vi "Parse VI Documentation String.vi"(7 "NOTE-Map":variant, 11 "Documentation":string) -> (0 "Ctrl-Doc Map":variant, 1 "Control Docs":cluster{"filtered array":string[]}[](array[cluster]), 2 "Core Doc":string, 3 "Documentation (dup)":string)   [LabVIEW 2017, in "csmdoc.lvlib"]
uses:
  csmdoc.lvlib
  Communicable State Machine.lvlib
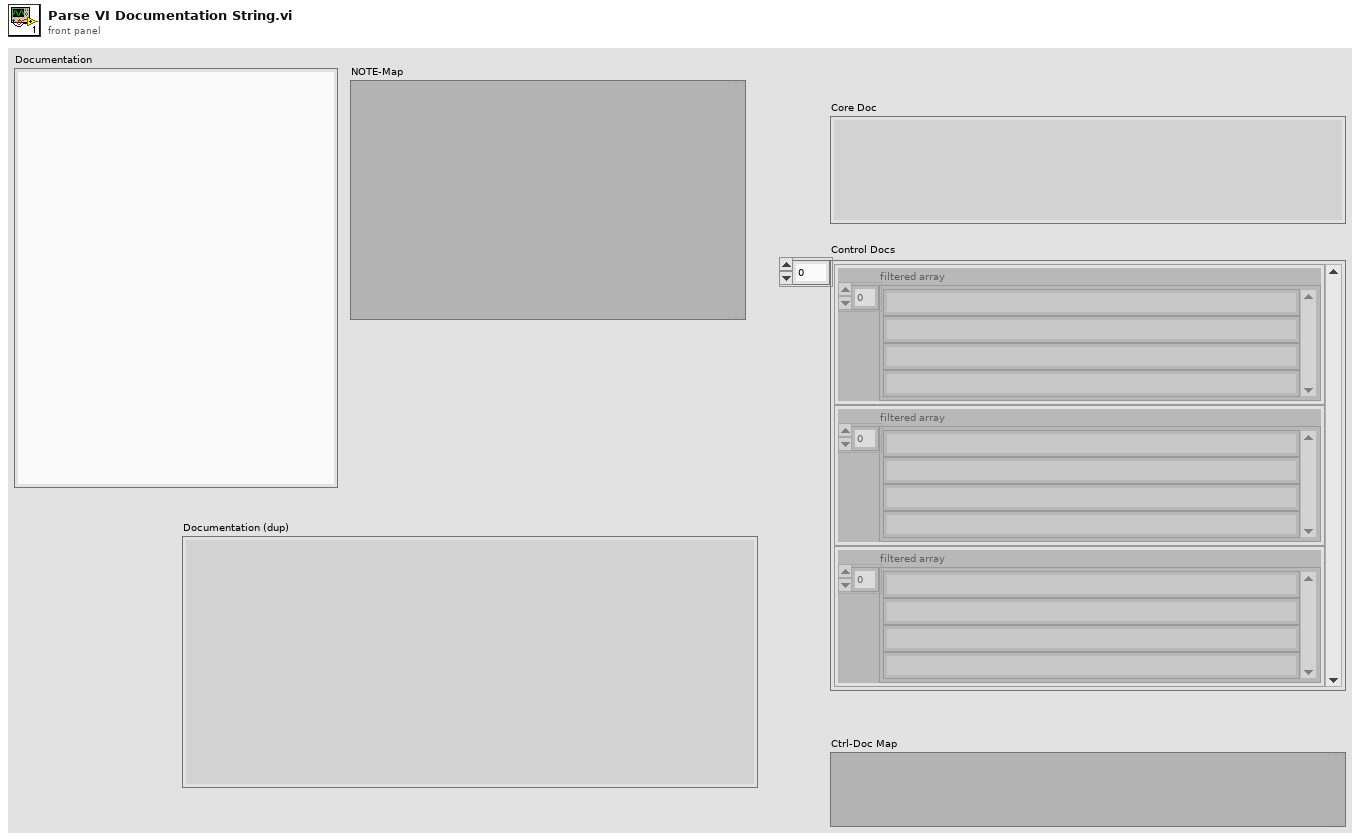
[diagram p1: front panel]
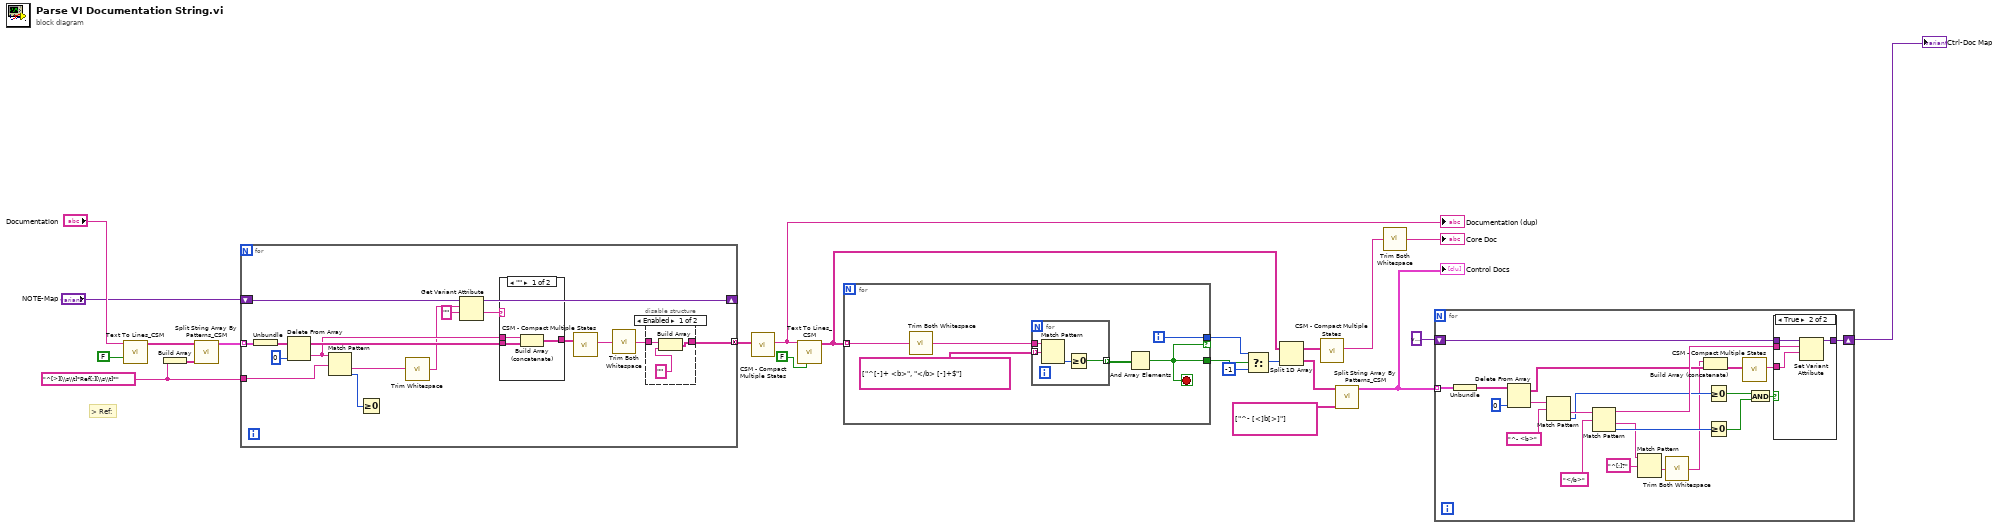
[diagram p0: block diagram]
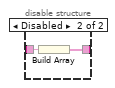
[diagram p2: hidden frame]
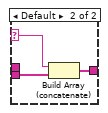
[diagram p3: hidden frame]
diagram:
  w6 = "^[>][\\s\\t]*Ref[:][\\s\\t]*" ("delimited string")
  # "> Ref:"
  n1 = call "Text To Lines_CSM.vi"("Remove Empty Lines?(T)"=FALSE, "string"="Documentation") -> ("Lines"=w8:string[])  [unwired: 8 in, 1 out]
  n2 = Build Array(w6) -> (w9:string[])
  n3 = call "Split String Array By Patterns_CSM.vi"("patterns"=w9, "Text Array"=w8) -> ("Array"=w7:cluster{"filtered array":string[]}[])  [unwired: 9 in]
  n4 = for {
    tunnel: w7 -> [w40] mode=indexing
    tunnel: w6 -> [w37]
    shift-right: [w33] -> _
    shift-left: "NOTE-Map" -> [w34]
    tunnel: [w31] -> w4 mode=concatenating
    n5 = Unbundle(w40) -> ("filtered array"=w39:string[])
    n6 = Delete From Array(array=w39, index=0) -> (deleted portion=w32:string, array with subset deleted=w35:string[])  [unwired: 1 in]
    n7 = Match Pattern(string=w32, regular expression=w37) -> (after substring=w36:string, offset past match=w30:i32)  [unwired: 1 in, 2 out]
    n8 = Greater Or Equal To 0?(x=w30) -> ()  [unwired: 1 out]
    n9 = call <vilib>:"Trim Whitespace.vi"("string"=w36) -> ("trimmed string"=w29:string)  [unwired: 1 in]
    n10 = Get Variant Attribute(Variant=w34, name=w29, default value (empty Variant)="" ("delimited string")) -> (duplicate Variant=w33:variant, value=w25:string)  [unwired: 1 in, 2 out]
    n11 = case shown="\"\"" w25 {
      selector: w25 -> [_ w49]
      tunnel: w35 -> [w48 w51]
      tunnel: [w47 w50] -> w27
      tunnel: w32 -> [w46 _]
      frame "" {
        n12 = Build Array (concatenate)(w46, w48) -> (w47:string[])
      }
      frame Default {
        n13 = Build Array (concatenate)(w49, w51) -> (w50:string[])
      }
    }
    n14 = call "CSM - Compact Multiple States.vi"("Multiple States"=w27) -> ("States"=w26:string)  [unwired: 9 in]
    n15 = call "Trim Both Whitespace.vi"("string"=w26) -> ("trimmed string"=w24:string)  [unwired: 1 in]
    n16 = disable-structure shown="Enabled" {
      disable-tunnel: w24 -> [w43 w45]
      disable-tunnel: [w42 w44] -> w31
      frame Enabled {
        n17 = Build Array(w43, "" ("delimited string")) -> (w42:string[])
      }
      frame Disabled {
        n18 = Build Array(w45) -> (w44:string[])
      }
    }
  }
  n19 = call "CSM - Compact Multiple States.vi"("Multiple States"=w4) -> ("States"=w3:string)  [unwired: 9 in]
  "Documentation (dup)" <- w3
  n20 = call "Text To Lines_CSM.vi"("Remove Empty Lines?(T)"=FALSE, "string"=w3) -> ("Lines"=w15:string[])  [unwired: 8 in, 1 out]
  n21 = for {
    tunnel: w15 -> [w57] mode=indexing
    tunnel: [w54] -> w13 if=w52
    tunnel: [w52] -> w12
    i -> [w54]
    stop <- w52 stop-if-true
    n22 = call "Trim Both Whitespace.vi"("string"=w57) -> ("trimmed string"=w55:string)  [unwired: 1 in]
    n23 = for {
      tunnel: string[] ["^[-]+ <b>", "</b> [-]+$"] ("regular expression") -> [w61] mode=indexing
      tunnel: w55 -> [w60]
      tunnel: [w58] -> w53 mode=indexing
      n24 = Match Pattern(string=w60, regular expression=w61) -> (offset past match=w59:i32)  [unwired: 1 in, 3 out]
      n25 = Greater Or Equal To 0?(x=w59) -> (x >= 0?=w58:bool)
    }
    n26 = And Array Elements(Boolean array=w53) -> (logical AND=w52:bool)
  }
  n27 = Select(t=w13, s=w12, f=-1) -> (s? t:f=w16:i32)
  n28 = Split 1D Array(array=w15, index=w16) -> (first subarray=w22:string[], second subarray=w17:string[])
  n29 = call "CSM - Compact Multiple States.vi"("Multiple States"=w22) -> ("States"=w11:string)  [unwired: 9 in]
  n30 = call "Split String Array By Patterns_CSM.vi"("patterns"=string[] ["^- [<]b[>]"], "Text Array"=w17) -> ("Array"=w19:cluster{"filtered array":string[]}[])  [unwired: 9 in]
  "Control Docs" <- w19
  n31 = call "Trim Both Whitespace.vi"("string"=w11) -> ("trimmed string"=→"Core Doc":string)  [unwired: 1 in]
  n32 = for {
    tunnel: w19 -> [w83] mode=indexing
    shift-right: [w75] -> w21
    shift-left: variant -> [w76]
    n33 = Unbundle(w83) -> ("filtered array"=w82:string[])
    n34 = Delete From Array(array=w82, index=0) -> (deleted portion=w80:string, array with subset deleted=w68:string[])  [unwired: 1 in]
    n35 = Match Pattern(string=w80, regular expression="^- <b>" ("delimited string")) -> (after substring=w78:string, offset past match=w72:i32)  [unwired: 1 in, 2 out]
    n36 = Match Pattern(string=w78, regular expression="</b>" ("delimited string")) -> (before substring=w74:string, after substring=w65:string, offset past match=w71:i32)  [unwired: 1 in, 1 out]
    n37 = Match Pattern(string=w65, regular expression="^[:]?") -> (after substring=w63:string)  [unwired: 1 in, 3 out]
    n38 = call "Trim Both Whitespace.vi"("string"=w63) -> ("trimmed string"=w62:string)  [unwired: 1 in]
    n39 = Build Array (concatenate)(w62, w68) -> (w66:string[])
    n40 = Greater Or Equal To 0?(x=w72) -> (x >= 0?=w70:bool)
    n41 = Greater Or Equal To 0?(x=w71) -> (x >= 0?=w69:bool)
    n42 = call "CSM - Compact Multiple States.vi"("Multiple States"=w66) -> ("States"=w67:string)  [unwired: 9 in]
    n43 = And(x=w70, y=w69) -> (x .and. y?=w73:bool)
    n44 = case shown="True" w73 {
      tunnel: w76 -> [w84 w88]
      tunnel: [w84 w87] -> w75
      tunnel: w74 -> [_ w86]
      tunnel: w67 -> [_ w85]
      frame False {
      }
      frame True {
        n45 = Set Variant Attribute(Variant=w88, name=w86, value=w85) -> (Variant out=w87:variant)  [unwired: 1 in, 2 out]
      }
    }
  }
  "Ctrl-Doc Map" <- w21
